vi "HexToWord.vi"(11 "数组":u16[](array[numeric]) format="%04xH") -> (3 "WORD":u16[](array[numeric]))   [LabVIEW 2016, in "总氮.lvlib"]
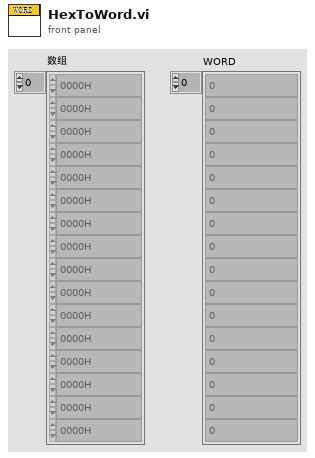
[diagram p1: front panel]
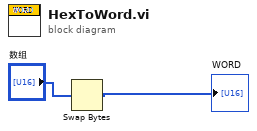
[diagram p0: block diagram]
diagram:
  n1 = Swap Bytes(anything="数组") -> (byte swapped=→"WORD":u16[])
